vi "iXon_Init_Cool.vi"(8 "error in (no error)":errorcluster, 9 "CoolToTargetTemp":bool=TRUE, 10 "Exposure Time (secs)":sgl=0.05 format="%.2f", 11 "Set Temp":i32=-60) -> (0 "error out":errorcluster, 1 "Current Temp":i32, 2 "Detector Y Pixels":i32, 3 "Detector X Pixels":i32)   [LabVIEW 2018]
panel:
  in  "Trigger":u32(ring) items=["Internal", "External"]
  out "Return from Initialize":u32
  # "Initialize iXon EMCCD with a few default settings, and cool to stable or target temperature"
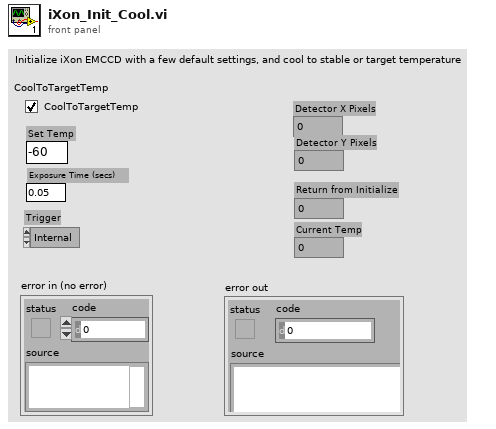
[diagram p1: front panel]
types:
  T1 = typedef "Error Code Enum typedef.ctl" = enum32{"N/A (0)", "DRV_ERROR_CODES", "DRV_SUCCESS", "DRV_VXDNOTINSTALLED", "DRV_ERROR_SCAN", "DRV_ERROR_CHECK_SUM", "DRV_ERROR_FILELOAD", "DRV_UNKNOWN_FUNC", "DRV_ERROR_VXD_INIT", "DRV_ERROR_ADDRESS", "DRV_ERROR_PAGELOCK", "DRV_ERROR_PAGEUNLOCK", "DRV_ERROR_BOARDTEST", "DRV_ERROR_ACK", "DRV_ERROR_UP_FIFO", "DRV_ERROR_PATTERN", "N/A (16)", "DRV_ACQUISITION_ERRORS", "DRV_ACQ_BUFFER", "DRV_ACQ_DOWNFIFO_FULL", "DRV_PROC_UNKONWN_INSTRUCTION", "DRV_ILLEGAL_OP_CODE", "DRV_KINETIC_TIME_NOT_MET", "DRV_ACCUM_TIME_NOT_MET", "DRV_NO_NEW_DATA", "N/A (25)", "DRV_SPOOLERROR", "N/A (27)", "N/A (28)", "N/A (29)", "N/A (30)", "N/A (31)", "N/A (32)", "DRV_TEMPERATURE_CODES", "DRV_TEMPERATURE_OFF", "DRV_TEMPERATURE_NOT_STABILIZED", "DRV_TEMPERATURE_STABILIZED", "DRV_TEMPERATURE_NOT_REACHED", "DRV_TEMPERATURE_OUT_RANGE", "DRV_TEMPERATURE_NOT_SUPPORTED", "DRV_TEMPERATURE_DRIFT", "N/A (41)", "N/A (42)", "N/A (43)", "N/A (44)", "N/A (45)", "N/A (46)", "N/A (47)", "N/A (48)", "DRV_GENERAL_ERRORS", "DRV_INVALID_AUX", "DRV_COF_NOTLOADED", "DRV_FPGAPROG", "DRV_FLEXERROR", "DRV_GPIBERROR", "N/A (55)", "N/A (56)", "N/A (57)", "N/A (58)", "N/A (59)", "N/A (60)", "N/A (61)", "N/A (62)", "N/A (63)", "DRV_DATATYPE", "DRV_DRIVER_ERRORS", "DRV_P1INVALID", "DRV_P2INVALID", "DRV_P3INVALID", "DRV_P4INVALID", "DRV_INIERROR", "DRV_COFERROR", "DRV_ACQUIRING", "DRV_IDLE", "DRV_TEMPCYCLE", "DRV_NOT_INITIALIZED", "DRV_P5INVALID", "DRV_P6INVALID", "DRV_INVALID_MODE", "DRV_INVALID_FILTER", "DRV_I2CERRORS", "DRV_I2CDEVNOTFOUND", "DRV_I2CTIMEOUT", "DRV_P7INVALID", "N/A (84)", "N/A (85)", "N/A (86)", "N/A (87)", "N/A (88)", "N/A (89)", "DRV_IOCERROR", "DRV_VRMVERSIONERROR"}
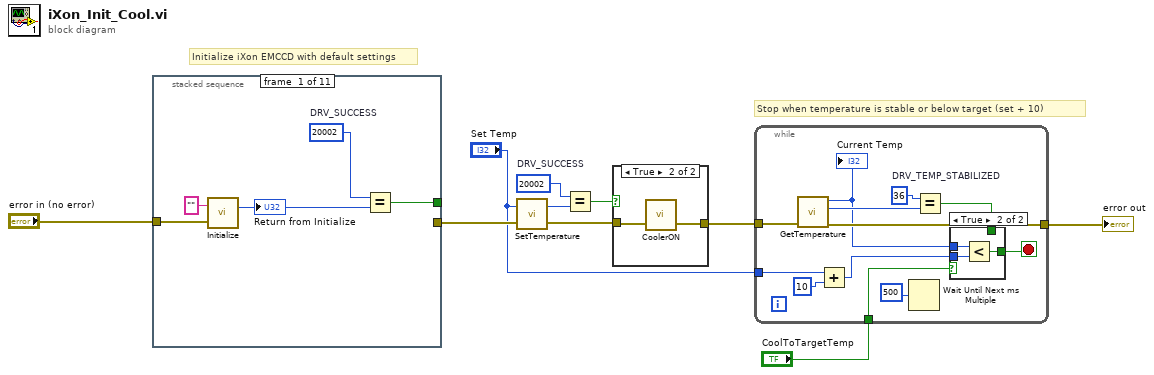
[diagram p0: block diagram]
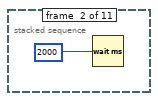
[diagram p4: hidden frame]
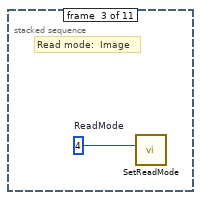
[diagram p5: hidden frame]
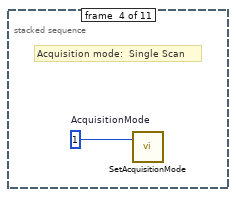
[diagram p6: hidden frame]
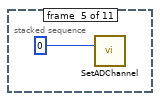
[diagram p7: hidden frame]
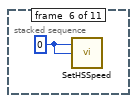
[diagram p8: hidden frame]
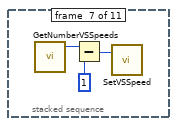
[diagram p9: hidden frame]
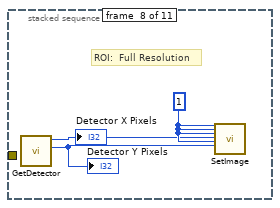
[diagram p10: hidden frame]
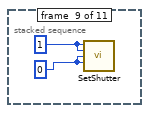
[diagram p11: hidden frame]
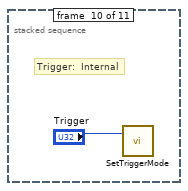
[diagram p12: hidden frame]
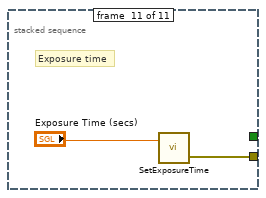
[diagram p13: hidden frame]
diagram:
  w8 = 20002  # DRV_SUCCESS
  # "Stop when temperature is stable or below target (set + 10)"
  # "Initialize iXon EMCCD with default settings"
  n1 = stacked-sequence {
    tunnel: [w13 _ _ _ _ _ _ _ _ _ _] -> _
    tunnel: "error in (no error)" -> [w12 _ _ _ _ _ _ _ _ _ _]
    tunnel: [_ _ _ _ _ _ _ _ _ _ w30] -> w7
    frame #0 {
      w11 = 20002  # DRV_SUCCESS
      n2 = call <userlib>:"Initialize.vi"("error in (no error)"=w12, "directory (\"\")"="" ("directory (\"\")")) -> ("DLL error code"=w15:u32)  [unwired: 1 out]
      "Return from Initialize" <- w15
      n3 = Equal?(x=w11, y=w15) -> (x = y?=w13:bool)
    }
    frame #1 {
      n4 = Wait (ms)(milliseconds to wait=u32 2000) -> ()  [unwired: 1 out]
    }
    frame #2 {
      w17 = u16 4  # ReadMode
      # "Read mode:  Image"
      n5 = call <userlib>:"SetReadMode.vi"("mode"=w17) -> ()  [unwired: 1 in, 2 out]
    }
    frame #3 {
      w18 = u16 1  # AcquisitionMode
      # "Acquisition mode:  Single Scan"
      n6 = call <userlib>:"SetAcquisitionMode.vi"("mode"=w18) -> ()  [unwired: 1 in, 2 out]
    }
    frame #4 {
      n7 = call <userlib>:"SetADChannel.vi"("channel"=0) -> ()  [unwired: 1 in, 2 out]
    }
    frame #5 {
      w20 = 0
      n8 = call <userlib>:"SetHSSpeed.vi"("index"=w20, "type"=w20) -> ()  [unwired: 2 in, 2 out]
    }
    frame #6 {
      n9 = call <userlib>:"GetNumberVSSpeeds.vi"() -> ("number"=w23:i32)  [unwired: 3 in, 2 out]
      n10 = Subtract(x=w23, y=1) -> (x-y=w21:i32)
      n11 = call <userlib>:"SetVSSpeed.vi"("index"=w21) -> ()  [unwired: 1 in, 2 out]
    }
    frame #7 {
      w26 = 1
      # "ROI:  Full Resolution"
      n12 = call <userlib>:"GetDetector.vi"() -> ("ypixels"=w25:i32, "xpixels"=w24:i32)  [unwired: 4 in, 2 out]
      "Detector Y Pixels" <- w25
      "Detector X Pixels" <- w24
      n13 = call <userlib>:"SetImage.vi"("hbin"=w26, "vbin"=w26, "hstart"=w26, "hend"=w24, "vstart"=w26, "vend"=w25) -> ()  [unwired: 20 in, 2 out]
    }
    frame #8 {
      w27 = 0
      w28 = 1
      n14 = call <userlib>:"SetShutter.vi"("type"=w28, "mode"=w28, "closingtime"=w27, "openingtime"=w27) -> ()  [unwired: 10 in, 2 out]
    }
    frame #9 {
      # "Trigger:  Internal"
      n15 = call <userlib>:"SetTriggerMode.vi"("mode"="Trigger") -> ()  [unwired: 1 in, 2 out]
    }
    frame #10 {
      # "Exposure time"
      n16 = call <userlib>:"SetExposureTime.vi"("time"="Exposure Time (secs)") -> ("error out"=w30:errorcluster)  [unwired: 1 in, 1 out]
    }
  }
  n17 = call <userlib>:"SetTemperature.vi"("error in (no error)"=w7, "temperature"="Set Temp") -> ("error out"=w5:errorcluster, "DLL error code"=w9:u32)
  n18 = Equal?(x=w8, y=w9) -> (x = y?=w6:bool)
  n19 = case shown="True" w6 {
    tunnel: w5 -> [w32 w34]
    tunnel: [w32 w33] -> w4
    frame False {
    }
    frame True {
      n20 = call <userlib>:"CoolerON.vi"("error in (no error)"=w34) -> ("error out"=w33:errorcluster)  [unwired: 1 in, 1 out]
    }
  }
  n21 = while {
    tunnel: [w44] -> w2
    tunnel: w4 -> [w40]
    tunnel: "Set Temp" -> [w38]
    tunnel: "CoolToTargetTemp" -> [w37]
    stop <- w36 stop-if-true
    w39 = 36  # DRV_TEMP_STABILIZED
    n22 = call <userlib>:"GetTemperature.vi"("error in (no error)"=w40) -> ("error out"=w44:errorcluster, "status"=w45:T1, "temperature"=w41:i32)  [unwired: 3 in, 1 out]
    "Current Temp" <- w41
    n23 = Add(x=w38, y=10) -> (x+y=w42:i32)
    n24 = Wait Until Next ms Multiple(millisecond multiple=u32 500) -> ()  [unwired: 1 out]
    n25 = Equal?(x=w39, y=w45) -> (x = y?=w35:bool)
    n26 = case shown="True" w37 {
      tunnel: w42 -> [_ w50]
      tunnel: w41 -> [_ w49]
      tunnel: [w47 w48] -> w36
      tunnel: w35 -> [w47 _]
      frame False {
      }
      frame True {
        n27 = Less?(x=w49, y=w50) -> (x < y?=w48:bool)
      }
    }
  }
  "error out" <- w2
